vi "保存文本文件.vi"() -> ()   [LabVIEW 2010]
panel:
  in  "stop":bool
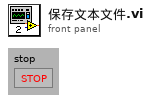
[diagram p1: front panel]
types:
  T1 = enum16{"open", "replace", "create", "open or create", "replace or create", "replace or create with confirmation"}
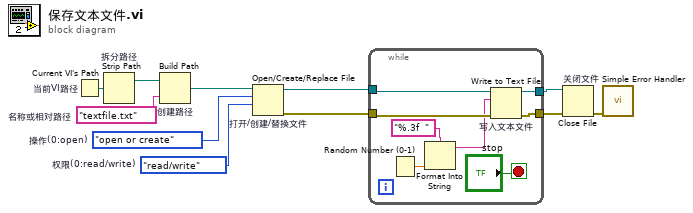
[diagram p0: block diagram]
diagram:
  w1 = enum16{"read/write", "read-only", "write-only"}."read/write"  # 权限(0:read/write)
  w2 = "textfile.txt"  # 名称或相对路径
  w3 = T1."open or create"  # 操作(0:open)
  n1 = Current VI's Path "当前VI路径"() -> (path=w11:path)
  n2 = Strip Path "拆分路径"(path=w11) -> (stripped path=w4:path)  [unwired: 1 out]
  n3 = Build Path "创建路径"(base path=w4, name or relative path=w2) -> (appended path=w10:path)
  n4 = Open/Create/Replace File "打开/创建/替换文件"(file path (use dialog)=w10, operation (0:open)=w3, access (0:read/write)=w1) -> (refnum out=w9:refnum<file>, error out=w8:errorcluster)  [unwired: 3 in, 1 out]
  n5 = while {
    tunnel: w9 -> [w15]
    tunnel: w8 -> [w14]
    tunnel: [w18] -> w7
    tunnel: [w17] -> w6
    stop <- "stop" stop-if-true
    n6 = Random Number (0-1)() -> (number: 0 to 1=w19:dbl)
    n7 = Format Into String(format string="%.3f  ", w19) -> (resulting string=w12:string)  [unwired: 2 in, 1 out]
    n8 = Write to Text File "写入文本文件"(file (use dialog)=w15, text=w12, error in=w14) -> (refnum out=w18:refnum<file>, error out=w17:errorcluster)  [unwired: 1 in, 1 out]
  }
  n9 = Close File "关闭文件"(refnum=w7, error in=w6) -> (error out=w5:errorcluster)  [unwired: 1 out]
  n10 = call <vilib>:"Simple Error Handler.vi"("error in (no error)"=w5) -> ()  [unwired: 4 in, 5 out]
